vi "setCurrentCmd.vi"(8 "error in (no error)":errorcluster, 9 "Data":variant, 10 "Name":string, 11 "Subsystem in":refnum<class "Subsystem.lvclass">) -> (0 "error out":errorcluster, 3 "Subsystem out":refnum<class "Subsystem.lvclass">)   [LabVIEW 2017, in "Subsystem.lvclass"]
uses:
  <userlib>/836-Library/Robot/Subsystem/Subsystem.lvclass
  <userlib>/836-Library/Robot/Command/Command.lvclass/Command.ctl
  <userlib>/836-Library/Robot/Subsystem/Subsystem.lvclass/Subsystem.ctl
  <userlib>/836-Library/Robot/Command/Command.lvclass
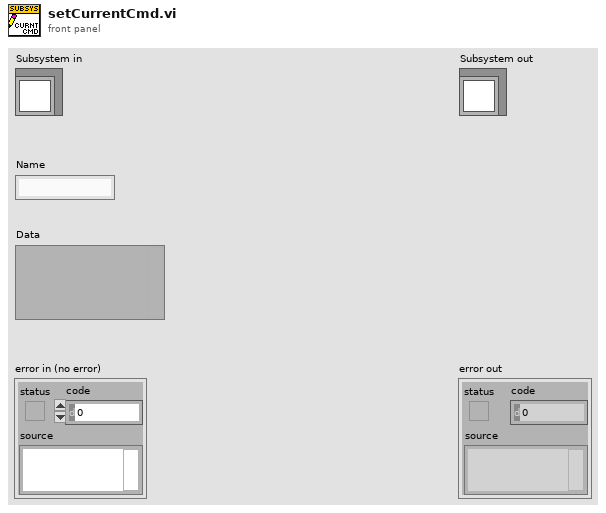
[diagram p1: front panel]
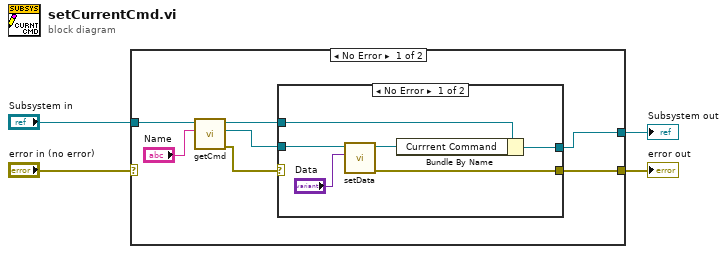
[diagram p0: block diagram]
diagram:
  n1 = case shown="No Error" "error in (no error)" {
    selector: "error in (no error)" -> [_ w20]
    tunnel: [w5 w20] -> w3
    tunnel: [w6 w21] -> w1
    tunnel: "Subsystem in" -> [w11 w21]
    frame No Error {
      n2 = call <userlib>:"getCmd.vi"("Name"="Name", "Subsystem in"=w11) -> ("error out"=w7:errorcluster, "Command"=w8:refnum<class "Command.lvclass">, "Subsystem out"=w9:refnum<class "Subsystem.lvclass">)  [unwired: 6 in, 1 out]
      n3 = case shown="No Error" w7 {
        selector: w7 -> [_ w18]
        tunnel: w9 -> [w15 w19]
        tunnel: w8 -> [w17 _]
        tunnel: [w13 w19] -> w6
        tunnel: [w12 w18] -> w5
        frame No Error {
          n4 = call <userlib>:"setData.vi"("Data"="Data", "Command in"=w17) -> ("error out"=w12:errorcluster, "Command out"=w14:refnum<class "Command.lvclass">)  [unwired: 8 in]
          n5 = Bundle By Name(cluster=w15, "Currrent Command"=w14) -> (w13:refnum<class "Subsystem.lvclass">)
        }
        frame Error {
        }
      }
    }
    frame Error {
    }
  }
  "error out" <- w3
  "Subsystem out" <- w1
